vi "Start Saw.vi"(8 "error in (no error)":errorcluster, 11 "Automation Controller in":refnum<class "Automation Controller.lvclass">) -> (0 "error out":errorcluster, 3 "State Machine Actor out":refnum<class "State Machine Actor.lvclass">)   [LabVIEW 2024, in "Automation Controller.lvlib" / "Automation Controller.lvclass"]
uses:
  Automation Controller.lvclass
  Automation Controller.lvclass/Automation Controller.ctl
  State Machine Actor/State Machine Actor/State Machine Actor.lvclass
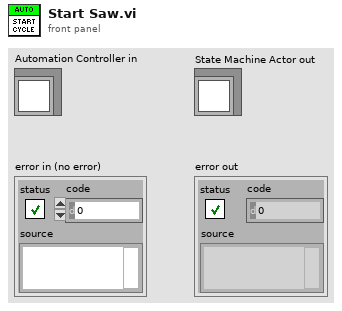
[diagram p1: front panel]
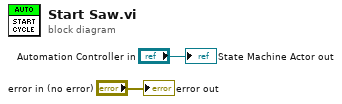
[diagram p0: block diagram]
diagram:
  "error out" <- "error in (no error)"
  "State Machine Actor out" <- "Automation Controller in"
